vi "Format Target Information.vi"(8 "error in":errorcluster, 11 "Targets Information":T1[](array[typedef]) {"Primary NIC"."IP Address Request Mode" items=["Static"=1, "DHCP/Link-Local"=2, "Link-Local Only"=4, "DHCP Only"=8]}) -> (0 "error out":errorcluster, 3 "Targets Information":string[][](array[string]))   [LabVIEW 2020]
uses:
  Controls/Target Information.ctl
  Controls/Target Network Settings.ctl
  Controls/System Credentials.ctl
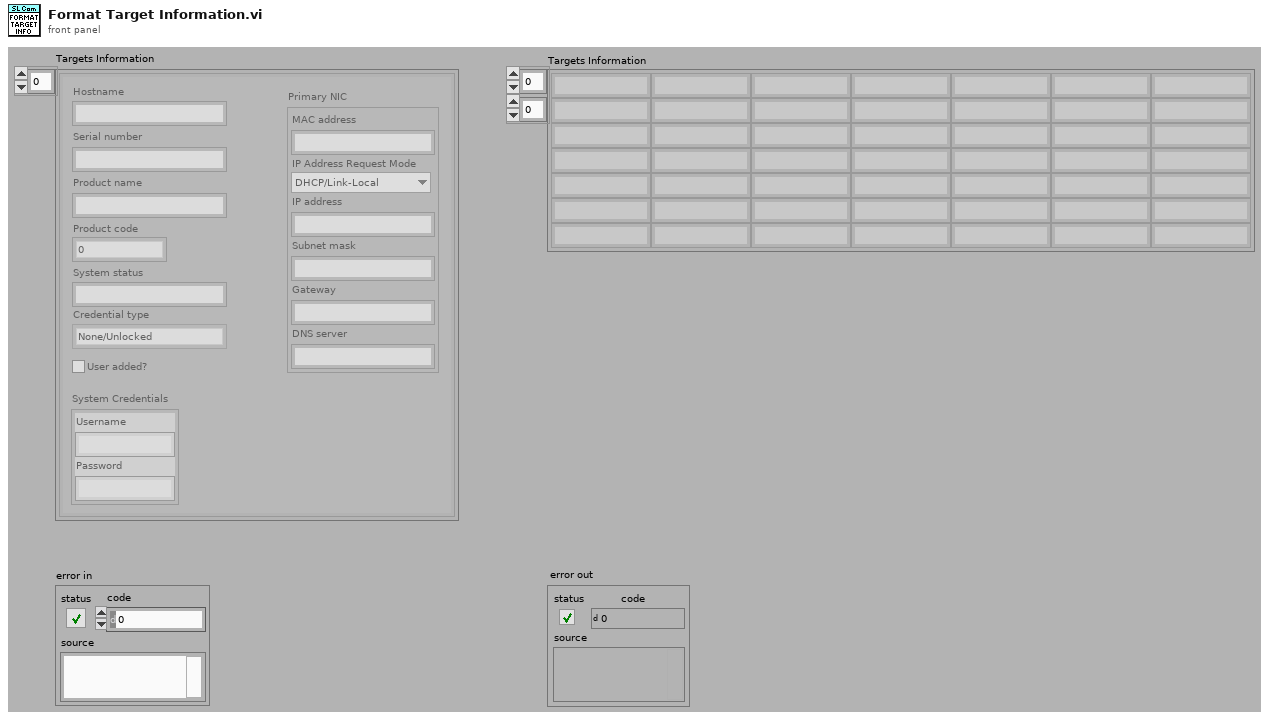
[diagram p1: front panel]
types:
  T1 = typedef "Target Information.ctl" = cluster{"Hostname":string, "Serial number":string, "Product name":string, "Product code":i32, "System status":string, "Credential type":enum16{"None/Unlocked", "FTP Password", "NIAuth Credentials"}, "User added?":bool, "Primary NIC":T2, "System Credentials":T3}
  T2 = typedef "Target Network Settings.ctl" = cluster{"MAC address":string, "IP Address Request Mode":i32, "IP address":string, "Subnet mask":string, "Gateway":string, "DNS server":string}
  T3 = typedef "System Credentials.ctl" = cluster{"Username":string, "Password":string}
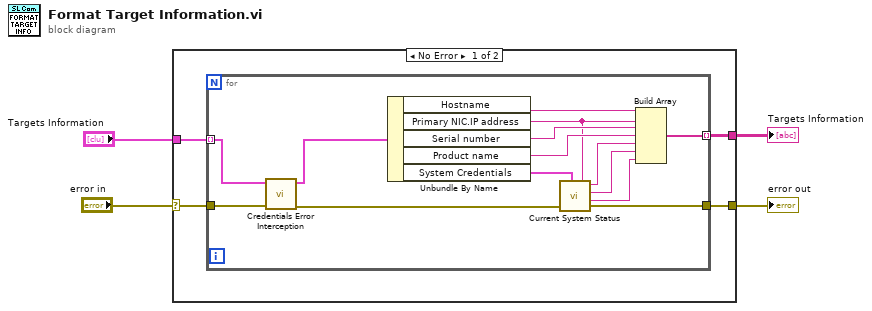
[diagram p0: block diagram]
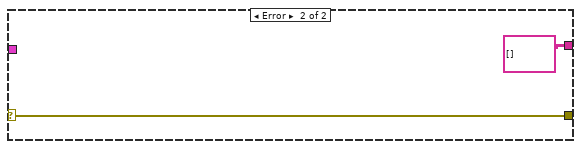
[diagram p2: hidden frame]
diagram:
  n1 = case shown="No Error" "error in" {
    selector: "error in" -> [w5 w24]
    tunnel: [w8 string[][] []] -> w4
    tunnel: "Targets Information" -> [w7 _]
    tunnel: [w6 w24] -> w2
    frame No Error {
      n2 = for {
        tunnel: w7 -> [w12] mode=indexing
        tunnel: [w20] -> w8 mode=indexing
        tunnel: w5 -> [w11]
        tunnel: [w17] -> w6
        n3 = call "Credentials Error Interception.vi"("error in"=w11, "Target settings in"=w12) -> ("error out"=w10:errorcluster, "Target settings out"=w9:T1)  [unwired: 8 in]
        n4 = Unbundle By Name(w9) -> ("Hostname"=w22:string, "Primary NIC.IP address"=w18:string, "Serial number"=w19:string, "Product name"=w21:string, "System Credentials"=w13:T3)
        n5 = call "Current System Status.vi"("System Credentials"=w13, "error in"=w10, "IP address"=w18) -> ("error out"=w17:errorcluster, "Requires Update?"=w14:string, "ImageTitle"=w15:string, "Firmware Version"=w16:string)  [unwired: 5 in]
        n6 = Build Array(w22, w18, w19, w21, w16, w15, w14) -> (w20:string[])
      }
    }
    frame Error {
    }
  }
  "Targets Information" <- w4
  "error out" <- w2
